vi "Test Test Fail if Expected API Call not Made.vi"(8 "error in (no error)":errorcluster, 11 "Test Case In":refnum<class "Mock Test.lvclass">) -> (0 "error out":errorcluster, 3 "Test Case Out":refnum<class "Mock Test.lvclass">)   [LabVIEW 2020, in "Mock Test.lvclass"]
uses:
  Mock Test.lvclass
  C:/Program Files (x86)/National Instruments/LabVIEW 2020/vi.lib/Astemes/LUnit/Test Case.lvclass
  <vilib>/Astemes/LUnit/Test Case.lvclass
  <vilib>/Astemes/LUnit/Test Case.lvclass/Test Case.ctl
  6053ebfb-fa78-43cc-b4be-896e65d0506d.vi
  <vilib>/Astemes/LUnit/Append Pass Result.vi
  <vilib>/Astemes/LUnit/Append Fail Result.vi
  <vilib>/Astemes/LUnit/Describe Comparison.vi
  <vilib>/Astemes/LUnit/Compare Variants.vi
  <vilib>/Astemes/LUnit/Variant to string.vi
  <vilib>/Utility/Data Type/Get Type Information.vi
  <vilib>/Utility/LVClass/Get LV Class Name.vi
  Mock/Mock.lvclass
  One Of/One Of.lvclass
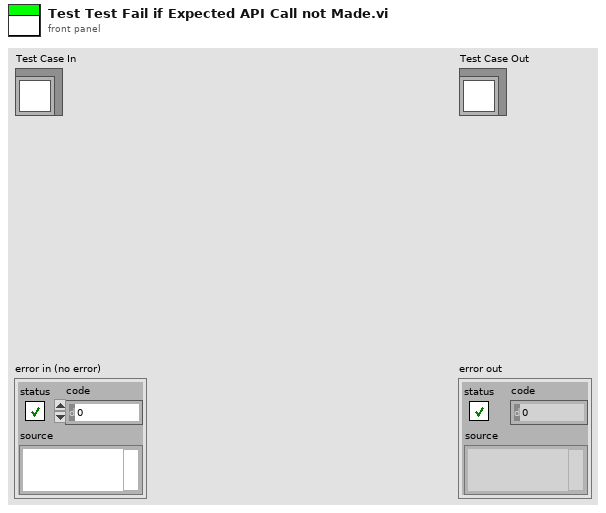
[diagram p1: front panel]
types:
  T1 = enum16{"", "Passed", "Failed", "Error", "Skipped", "Setup Error", "Broken", "Teardown Error"}
  T2 = cluster{"Name":string, "Message":string, "Description":string, "Status":enum16{"", "Passed", "Failed", "Error", "Skipped", "Setup Error", "Broken", "Teardown Error"}, "Result Type":enum16{"Test Case", "Test Suite", "Test Run", "Pass", "Fail", "Skip", "Pass if", "Fail if", "Pass if Error", "Fail if Error", "Pass if Equal", "Fail if Equal"}, "Execution Time":dbl}[]
  T3 = cluster{"Name":string, "Message":string, "Description":string, "Status":enum16{"", "Passed", "Failed", "Error", "Skipped", "Setup Error", "Broken", "Teardown Error"}, "Result Type":enum16{"Test Case", "Test Suite", "Test Run", "Pass", "Fail", "Skip", "Pass if", "Fail if", "Pass if Error", "Fail if Error", "Pass if Equal", "Fail if Equal"}, "Execution Time":dbl}
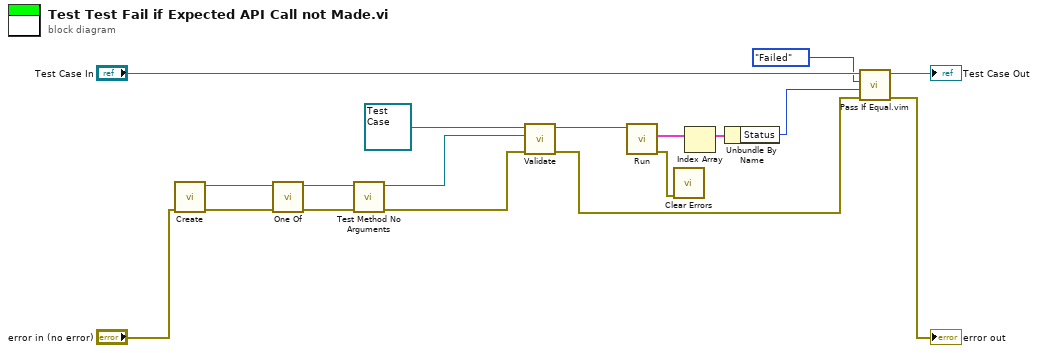
[diagram p0: block diagram]
diagram:
  n1 = call "Create.vi"("error in (no error)"="error in (no error)") -> ("error out"=w17:errorcluster, "Mock Out"=w18:refnum<class "Mock.lvclass">)  [unwired: 9 in]
  n2 = call "One Of.vi"("error in (no error)"=w17, "Mock in"=w18) -> ("error out"=w15:errorcluster, "Mock out"=w16:refnum<class "Mock.lvclass">)  [unwired: 8 in]
  n3 = call-dynamic "Test Method No Arguments.vi"("error in (no error)"=w15, "Mock In"=w16) -> ("error out"=w13:errorcluster, "Mock Out"=w14:refnum<class "Mock.lvclass">)  [unwired: 8 in]
  n4 = call "Validate.vi"("error in (no error)"=w13, "Mock.lvclass"=w14, "LUnit Test Case In"=refnum<class "Test Case.lvclass"> refnum) -> ("error out"=w12:errorcluster, "LUnit Test Case Out"=w6:refnum<class "Test Case.lvclass">)  [unwired: 7 in]
  n5 = call-dynamic "Run.vi"("LUnit Test Case In"=w6) -> ("error out"=w1:errorcluster, "Results"=w5:T2)  [unwired: 7 in, 2 out]
  n6 = call <vilib>:"Clear Errors.vi"("error in (no error)"=w1) -> ()  [unwired: 5 in, 2 out]
  n7 = Index Array(array=w5) -> (element=w4:T3)  [unwired: 1 in]
  n8 = Unbundle By Name(w4) -> ("Status"=w3:T1)
  n9 = call "Pass If Equal.vim"("error in (no error)"=w12, "Actual"=w3, "Expected"=T1."Failed" ("Status"), "LUnit Test Case In"="Test Case In") -> ("error out"=→"error out":errorcluster, "LUnit Test Case Out"=→"Test Case Out":refnum<class "Mock Test.lvclass">)  [unwired: 6 in]
